vi "Write listener ID.vi"(8 "error in (no error)":errorcluster, 10 "listener ID":refnum<k5>, 11 "WebSocket Service Actor in":refnum<class "WebSocket Service Actor.lvclass">) -> (0 "error out":errorcluster, 3 "WebSocket Service Actor out":refnum<class "WebSocket Service Actor.lvclass">)   [LabVIEW 2016]
uses:
  WebSocket Service Actor.lvclass
  C:/Program Files (x86)/National Instruments/LabVIEW 2016/vi.lib/ActorFramework/Actor/Actor.lvclass
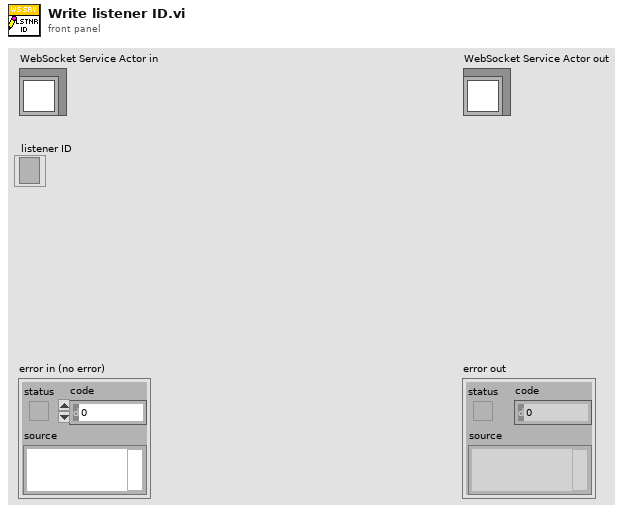
[diagram p1: front panel]
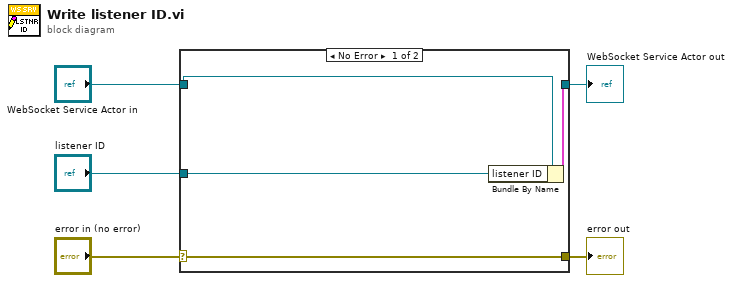
[diagram p0: block diagram]
diagram:
  n1 = case shown="No Error" "error in (no error)" {
    selector: "error in (no error)" -> [w9 w10]
    tunnel: [w9 w10] -> w4
    tunnel: [w7 w11] -> w2
    tunnel: "WebSocket Service Actor in" -> [w8 w11]
    tunnel: "listener ID" -> [w6 _]
    frame No Error {
      n2 = Bundle By Name(cluster=w8, "listener ID"=w6) -> (w7:cluster{})
    }
    frame Error {
    }
  }
  "error out" <- w4
  "WebSocket Service Actor out" <- w2
